vi "Close Monitor.vi"(8 "error in (no error)":errorcluster, 11 "VI Refnum":refnum<vi>) -> (0 "error out":errorcluster)   [LabVIEW 2018, in "Process Bar.lvclass"]
uses:
  Process Bar.lvclass
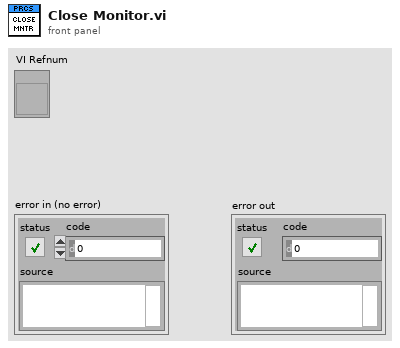
[diagram p1: front panel]
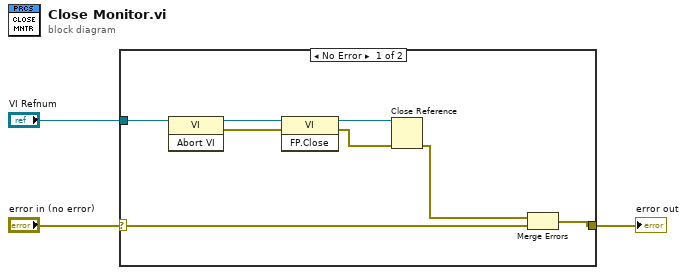
[diagram p0: block diagram]
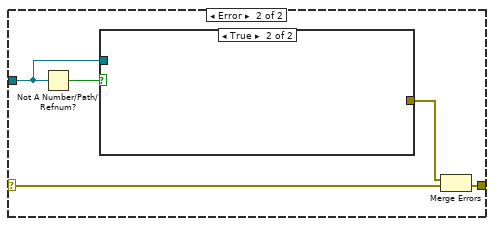
[diagram p2: hidden frame]
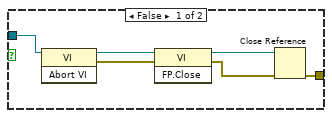
[diagram p3: hidden frame]
diagram:
  n1 = case shown="No Error" "error in (no error)" {
    selector: "error in (no error)" -> [w4 w14]
    tunnel: "VI Refnum" -> [w11 w15]
    tunnel: [w5 w12] -> w2
    frame No Error {
      n2 = invoke class="VI" method="Abort VI"(reference=w11) -> (reference out=w10:refnum<vi>, error out=w9:errorcluster)  [unwired: 2 in, 1 out]
      n3 = invoke class="VI" method="FP.Close"(reference=w10, error in=w9) -> (reference out=w8:refnum<vi>, error out=w7:errorcluster)  [unwired: 1 in, 1 out]
      n4 = Close Reference(reference=w8, error in (no error)=w7) -> (error out=w6:errorcluster)
      n5 = Merge Errors(w6, w4) -> (w5:errorcluster)
    }
    frame Error {
      n6 = Not A Number/Path/Refnum?(number/path/refnum=w15) -> (NaN/Path/Refnum?=w16:bool)
      n7 = case shown="True" w16 {
        tunnel: w15 -> [w18 _]
        tunnel: [w17 _] -> w13
        frame False {
          n8 = invoke class="VI" method="Abort VI"(reference=w18) -> (reference out=w22:refnum<vi>, error out=w21:errorcluster)  [unwired: 2 in, 1 out]
          n9 = invoke class="VI" method="FP.Close"(reference=w22, error in=w21) -> (reference out=w20:refnum<vi>, error out=w19:errorcluster)  [unwired: 1 in, 1 out]
          n10 = Close Reference(reference=w20, error in (no error)=w19) -> (error out=w17:errorcluster)
        }
        frame True {
        }
      }
      n11 = Merge Errors(w13, w14) -> (w12:errorcluster)
    }
  }
  "error out" <- w2
